vi "generate table.vi"(5 "to cvt":refnum<vi>, 6 "Direction":enum32{"From CVT", "To CVT"}(radio), 7 "from cvt":refnum<vi>, 8 "error in":errorcluster, 9 "avail tags":refnum<vi>, 10 "engine configuration in":refnum<class "engine configuration.lvclass">, 11 "cvt in":refnum<class "CVT configuration.lvclass">) -> (0 "error out":errorcluster, 3 "cvt out":refnum<class "CVT configuration.lvclass">)   [LabVIEW 2013, in "CVT editor node.lvclass"]
uses:
  CVT editor node.lvclass
  configuration/CVT configuration.lvclass
  <vilib>/NI/Module Execution Interface/Engine Configuration/engine configuration.lvclass
  <vilib>/NI/Configuration Framework/serializable configuration/NISE_CEF_serializable configuration.lvclass/NISE_CEF_serializable configuration.ctl
  configuration/CVT configuration.lvclass/CVT configuration.ctl
  <vilib>/NI/Tag Bus/tag/tag descriptor.lvclass/tag descriptor.ctl
  <vilib>/NI/Tag Bus Module Framework/channel/channel classification.ctl
  <vilib>/NI/Tag Bus Module Framework/channel/TBM channel.lvclass/TBM channel.ctl
  <vilib>/NI/Module Execution Interface/Engine Configuration/engine configuration.lvclass/engine configuration.ctl
  <vilib>/NI/Tag Bus/tag/read tag name.vi
  <vilib>/NI/Tag Bus Module Framework/channel/Read channel classification.vi
  <vilib>/NI/Tag Bus/tag/read data type.vi
  <vilib>/NI/Configuration Framework/serializable configuration/Read UID.vi
  configuration/Read channels.vi
  <vilib>/Utility/LVClass/Get LV Class Name.vi
  <vilib>/NI/Configuration Framework/error generator.vi
  <vilib>/NI/Tag Bus Module Framework/channel/TBM channel.lvclass
  <vilib>/NI/Tag Bus/tag/tag descriptor.lvclass
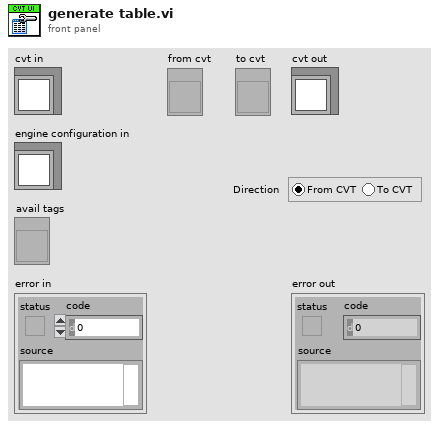
[diagram p1: front panel]
types:
  T1 = typedef "tag bus.lvlib/tag descriptor.lvclass/Data Type.ctl" = enum16{"Double", "Single", "I64", "I32", "I16", "I8", "U64", "U32", "U16", "U8", "Boolean", "String", "Array of Double", "Array of Single", "Array of I64", "Array of I32", "Array of I16", "Array of I8", "Array of U64", "Array of U32", "Array of U16", "Array of U8", "Array of Boolean", "Array of String"}
  T2 = typedef "TBM channel.lvclass/channel classification.ctl" = enum16{"input data", "output data", "processing parameter", "processing result"}
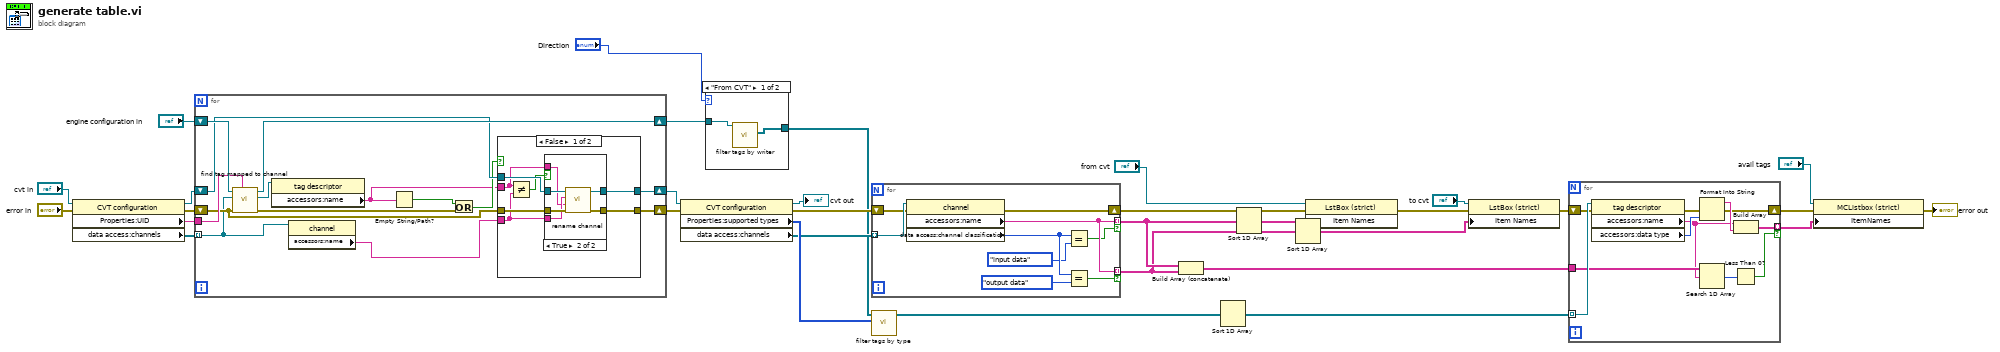
[diagram p0: block diagram]
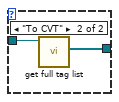
[diagram p2: hidden frame]
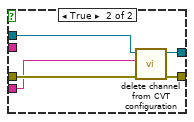
[diagram p4: hidden frame]
diagram:
  n1 = property class="CVT configuration"(reference="cvt in", error in="error in") -> (reference out=w30:refnum<class "CVT configuration.lvclass">, error out=w31:errorcluster, "Properties:UID"=w26:string, "data access:channels"=w32:refnum<class "TBM channel.lvclass">[])
  n2 = for {
    tunnel: w32 -> [w36] mode=indexing
    shift-right: [w44] -> w17
    shift-left: "engine configuration in" -> [w46]
    shift-right: [w41] -> w29
    shift-left: w30 -> [w39]
    tunnel: w26 -> [w45]
    shift-right: [w40] -> w28
    shift-left: w31 -> [w37]
    n3 = call <vilib>:"find tag mapped to channel.vi"("owner"=w45, "error in"=w37, "channel"=w36, "engine configuration in"=w46) -> ("error out"=w35:errorcluster, "tag"=w43:refnum<class "tag descriptor.lvclass">, "engine configuration out"=w44:refnum<class "engine configuration.lvclass">)  [unwired: 5 in]
    n4 = property class="tag descriptor"(reference=w43) -> ("accessors:name"=w33:string)  [unwired: 1 in, 2 out]
    n5 = property class="channel"(reference=w36) -> ("accessors:name"=w34:string)  [unwired: 1 in, 2 out]
    n6 = Empty String/Path?(string/path=w33) -> (empty?=w42:bool)
    n7 = Or(x=w42, y=w35) -> (x .or. y?=w38:bool)
    n8 = case shown="False" w38 {
      tunnel: [w50 w66] -> w41
      tunnel: [w53 w65] -> w40
      tunnel: w37 -> [w52 w64]
      tunnel: w39 -> [w51 w63]
      tunnel: w34 -> [w48 w62]
      tunnel: w33 -> [w47 _]
      frame False {
        n9 = Not Equal?(x=w47, y=w48) -> (x != y?=w49:bool)
        n10 = case shown="True" w49 {
          tunnel: [w55 w60] -> w53
          tunnel: w52 -> [w55 w61]
          tunnel: w51 -> [w54 w59]
          tunnel: [w54 w58] -> w50
          tunnel: w48 -> [_ w57]
          tunnel: w47 -> [_ w56]
          frame False {
          }
          frame True {
            n11 = call "rename channel.vi"("error in"=w61, "new name"=w56, "old name"=w57, "CVT configuration in"=w59) -> ("error out"=w60:errorcluster, "CVT configuration out"=w58:refnum<class "CVT configuration.lvclass">)  [unwired: 6 in]
          }
        }
      }
      frame True {
        n12 = call "delete channel from CVT configuration.vi"("error in"=w64, "channel to delete"=w62, "CVT configuration in"=w63) -> ("error out"=w65:errorcluster, "CVT configuration out"=w66:refnum<class "CVT configuration.lvclass">)  [unwired: 7 in]
      }
    }
  }
  n13 = property class="CVT configuration"(reference=w29, error in=w28) -> (reference out=→"cvt out":refnum<class "CVT configuration.lvclass">, error out=w24:errorcluster, "Properties:supported types"=w27:T1[], "data access:channels"=w25:refnum<class "TBM channel.lvclass">[])
  n14 = case shown="\"From CVT\"" "Direction" {
    tunnel: w17 -> [w68 w70]
    tunnel: [w67 w69] -> w16
    frame "From CVT" {
      n15 = call <vilib>:"filter tags by writer.vi"("engine configuration in"=w68) -> ("tag list"=w67:refnum<class "tag descriptor.lvclass">[])  [unwired: 9 in, 1 out]
    }
    frame "To CVT" {
      n16 = call <vilib>:"get full tag list.vi"("engine configuration in"=w70) -> ("tag list"=w69:refnum<class "tag descriptor.lvclass">[])  [unwired: 9 in, 1 out]
    }
  }
  n17 = for {
    tunnel: w25 -> [w79] mode=indexing
    shift-right: [w78] -> w10
    shift-left: w24 -> [w77]
    tunnel: [w76] -> w6 mode=indexing if=w74
    tunnel: [w76] -> w7 mode=indexing if=w73
    n18 = property class="channel"(reference=w79, error in=w77) -> (error out=w78:errorcluster, "accessors:name"=w76:string, "data access:channel classification"=w75:T2)  [unwired: 1 out]
    n19 = Equal?(x=w75, y=channel_classification."input data") -> (x = y?=w73:bool)
    n20 = Equal?(x=w75, y=channel_classification."output data") -> (x = y?=w74:bool)
  }
  n21 = call <vilib>:"filter tags by type.vi"("allowable types"=w27, "tags in"=w16) -> ("filtered tags"=w23:refnum<class "tag descriptor.lvclass">[])  [unwired: 9 in]
  n22 = Build Array (concatenate)(w7, w6) -> (w5:string[])
  n23 = Sort 1D Array(array=w23) -> (sorted array=w1:refnum<class "tag descriptor.lvclass">[])
  n24 = Sort 1D Array(array=w7) -> (sorted array=w3:string[])
  n25 = Sort 1D Array(array=w6) -> (sorted array=w2:string[])
  n26 = property class="LstBox (strict)"(reference="from cvt", error in=w10, "Item Names"=w3) -> (error out=w9:errorcluster)  [unwired: 1 out]
  n27 = property class="LstBox (strict)"(reference="to cvt", error in=w9, "Item Names"=w2) -> (error out=w22:errorcluster)  [unwired: 1 out]
  n28 = for {
    tunnel: w1 -> [w88] mode=indexing
    shift-right: [w85] -> w21
    shift-left: w22 -> [w87]
    tunnel: [w84] -> w20 mode=indexing if=w80
    tunnel: w5 -> [w83]
    n29 = property class="tag descriptor"(reference=w88, error in=w87) -> (error out=w86:errorcluster, "accessors:name"=w81:string, "accessors:data type"=w89:T1)  [unwired: 1 out]
    n30 = Format Into String(error in=w86, w89) -> (resulting string=w90:string, error out=w85:errorcluster)  [unwired: 2 in]
    n31 = Search 1D Array(1D array=w83, element=w81) -> (index of element=w82:i32)  [unwired: 1 in]
    n32 = Less Than 0?(x=w82) -> (x < 0?=w80:bool)
    n33 = Build Array(w81, w90) -> (w84:string[])
  }
  n34 = property class="MCListbox (strict)"(reference="avail tags", error in=w21, "ItemNames"=w20) -> (error out=→"error out":errorcluster)  [unwired: 1 out]
